vi "MPP.time.vi"(8 "error in (no error)":errorcluster, 10 "time":u16=2, 11 "VISA Refnum in":refnum<visa-resource-name>) -> (0 "error out":errorcluster, 3 "VISA Refnum out":refnum<visa-resource-name>)   [LabVIEW 2020, in "main.lvlib"]
uses:
  main.lvlib
  <instrlib>/HH PLA Series/HH PLA Series.lvlib
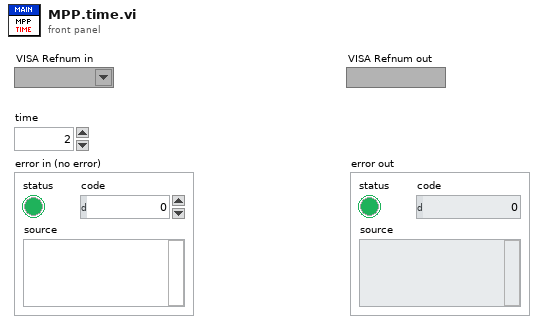
[diagram p1: front panel]
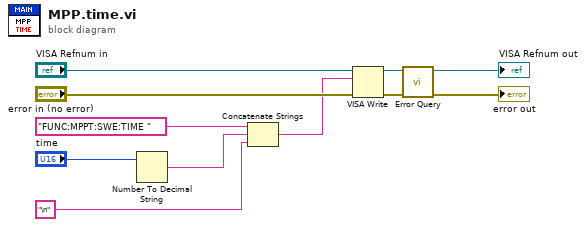
[diagram p0: block diagram]
diagram:
  n1 = Number To Decimal String(number="time") -> (decimal integer string=w3:string)  [unwired: 1 in]
  n2 = Concatenate Strings("FUNC:MPPT:SWE:TIME " ("write buffer"), w3, "\n") -> (w2:string)
  n3 = VISA Write(VISA resource name="VISA Refnum in", write buffer=w2, error in (no error)="error in (no error)") -> (VISA resource name out=w8:refnum<visa-resource-name>, error out=w9:errorcluster)  [unwired: 1 out]
  n4 = call <instrlib>:"Error Query.vi"("error in (no error)"=w9, "VISA resource name"=w8) -> ("error out"=→"error out":errorcluster, "VISA resource name out"=→"VISA Refnum out":refnum<visa-resource-name>)  [unwired: 6 in, 2 out]
